vi "Car Wash.vi"() -> ()   [LabVIEW 2013]
doc: "THis VI is a simulation of automated car wash controller.\nthe user can interact with the controls and indicator and select the car wash option and simulates the travel of the vehicle in the car wash.\n\nThe controller can perform these operation.\n- Indicate the car wash LED if the car wash is vacant or wash in progress.\n- Allow the user to select Wash option.\n- On pressing start the washing process will begin.\n- Indicator indicates the current wash process and display the elapsed time on indicator\n- Turn On the vehicle out of position LED and pause the elapsed time if the vehicle moves from its place \n during a cycle."
uses:
  Controls/Car Wash Indicators.ctl
  Controls/Wash Options.ctl
  Controls/Car wash cmd data cluster.ctl
  Controls/Car Wash States.ctl
  Controls/fgv.ctl
panel:
  in  "Start":bool
  out "Elapsed Time":dbl format="%0.2f"
  in  "stop":bool
  out "Wash Entry":bool
  in  "Wash Options":T1
  in  "Car Position Slider":u8(slide) max=3 scale=0.0..4.0
  out "Car Wash Indicators":T2
  # "Entry Console"
  # "Car Wash Display"
  # "Car Position Simulation"
  # "Pre-Soak\nH-P Wash\nL-P Wax\nSpot Free Rinse"
  # "Underbody Wash\nBug Remover"
  # "Tire Shine\nAir Dry"
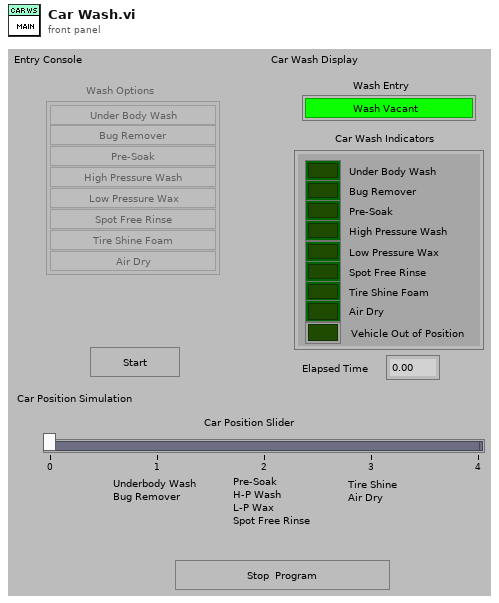
[diagram p1: front panel]
types:
  T1 = typedef "Wash Options.ctl" = cluster{"Underbody Wash":bool, "Bug Remover":bool, "Pre-Soak":bool, "High Pressure Wash":bool, "Low Pressure Wax":bool, "Spot Free Rinse":bool, "Tire Shine Foam":bool, "Air Dry":bool}
  T2 = typedef "Car Wash Indicators.ctl" = cluster{"Under Body Wash":bool, "Bug Remover":bool, "Pre-Soak":bool, "High Pressure Wash":bool, "Low Pressure Wax":bool, "Spot Free Rinse":bool, "Tire Shine Foam":bool, "Air Dry":bool, "Vehicle Out of Position":bool}
  T3 = typedef "Car wash cmd data cluster.ctl" = cluster{"Command":T4, "Data":variant}
  T4 = typedef "Car Wash States.ctl" = enum16{"Initialize", "Start1", "Start", "Underbody Wash", "Bug Remover", "Pre-Soak", "High Pressure Wash", "Low pressure wash", "Spot free Rinse", "Tire Shine Foam", "Air Dry", "Stop"}
  T5 = cluster{"Car Wash Indicators":T2, "Wash Entry":bool, "Elapsed TIme":dbl}
  T6 = enum8{"Enabled", "Disabled", "Disabled and Grayed Out"}
  T7 = typedef "fgv.ctl" = enum16{"Set Car Pos.", "Get Car Pos."}
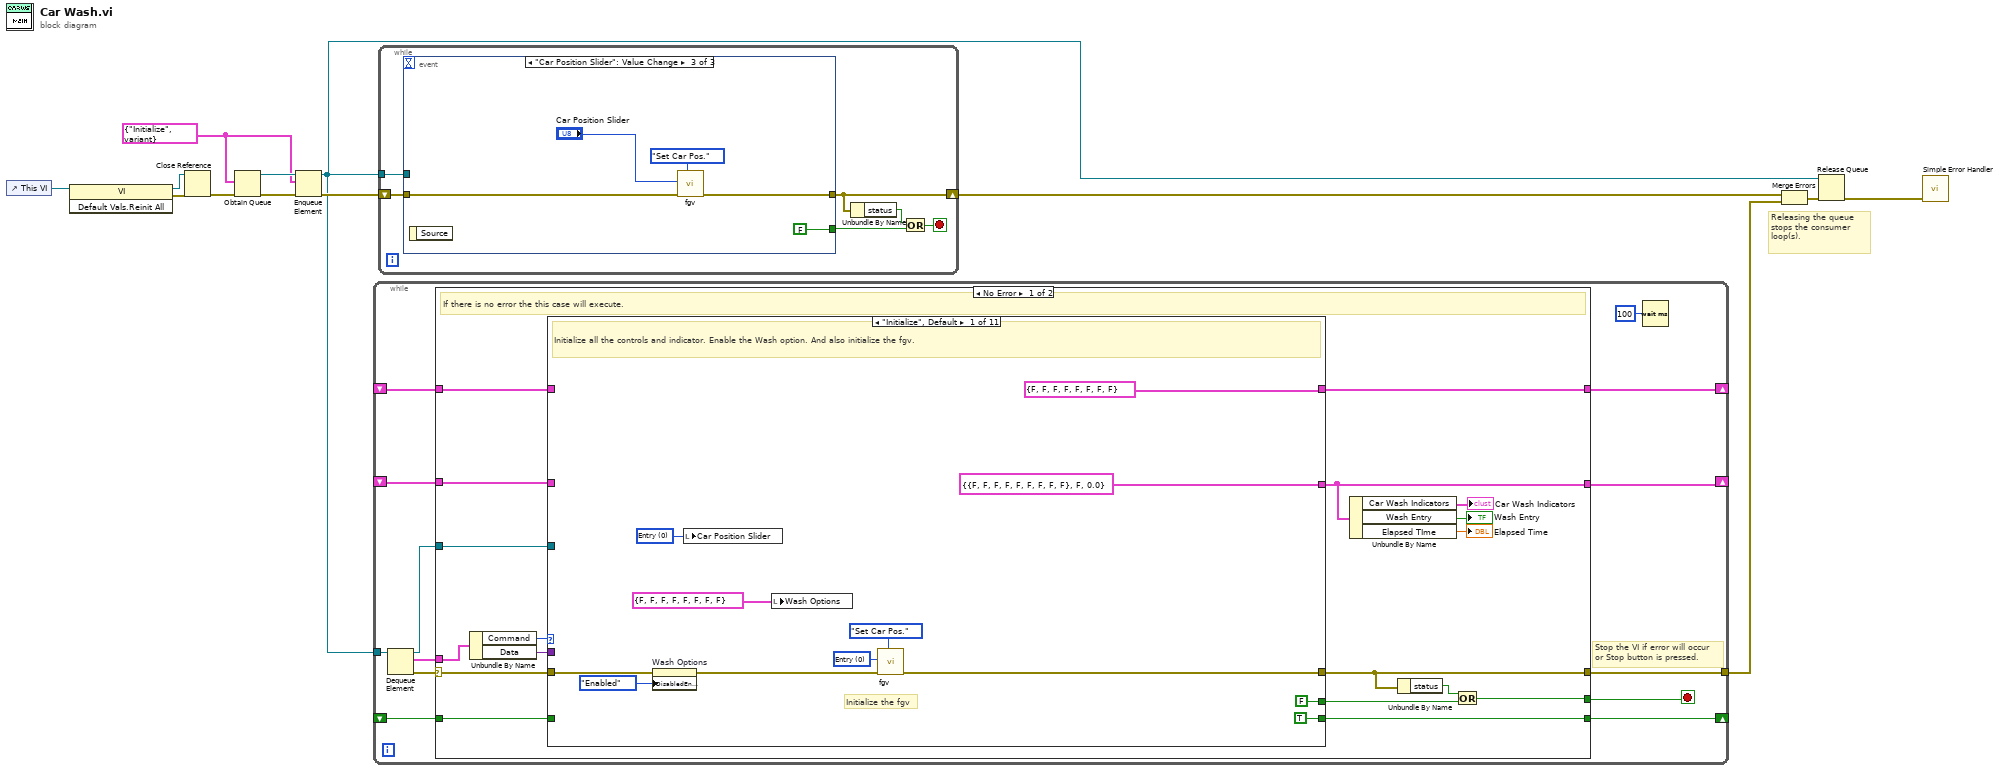
[diagram p0: block diagram]
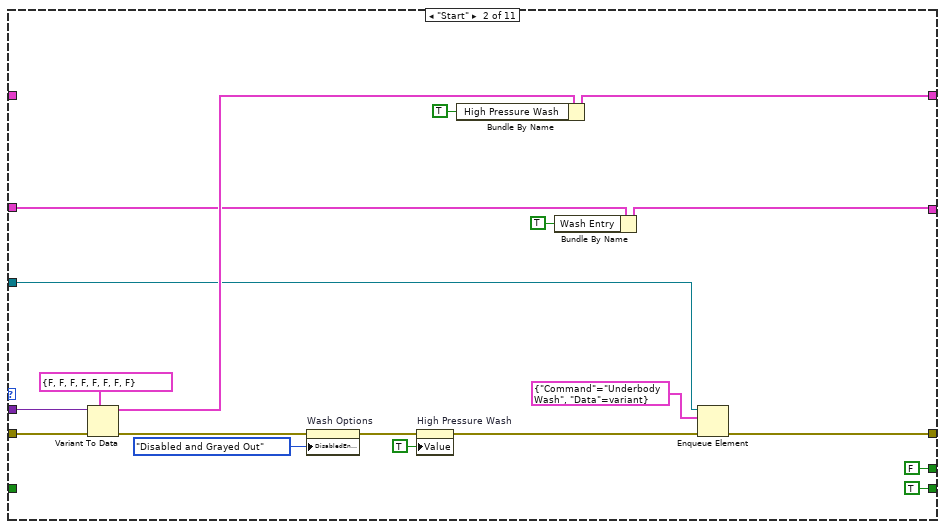
[diagram p2: hidden frame]
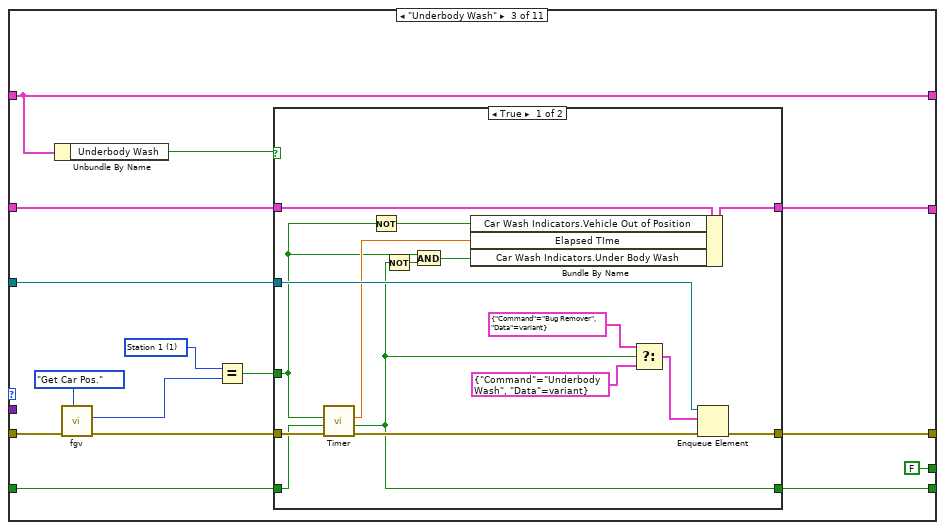
[diagram p3: hidden frame]
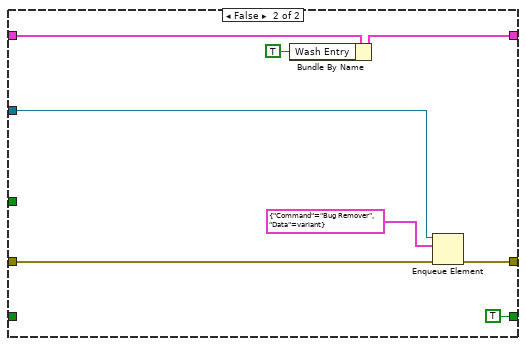
[diagram p4: hidden frame]
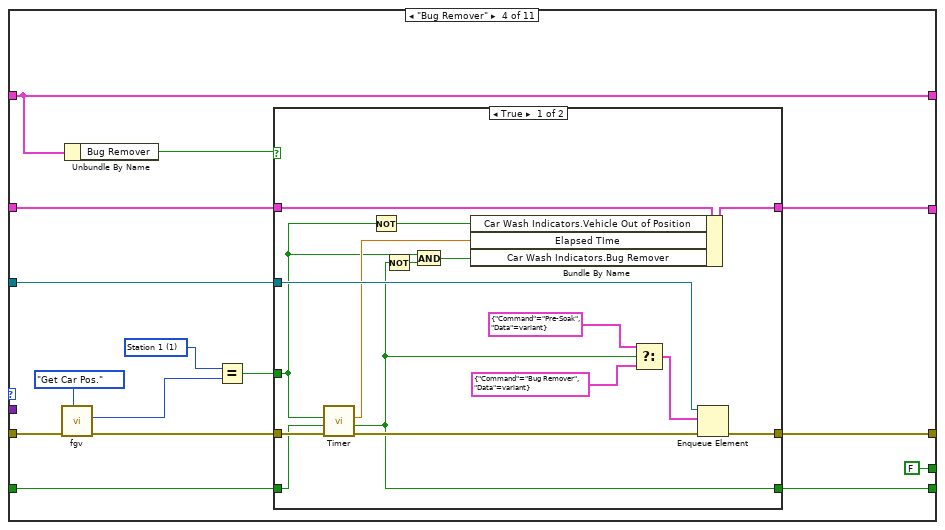
[diagram p5: hidden frame]
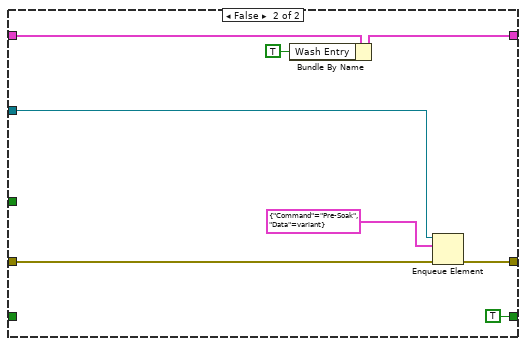
[diagram p6: hidden frame]
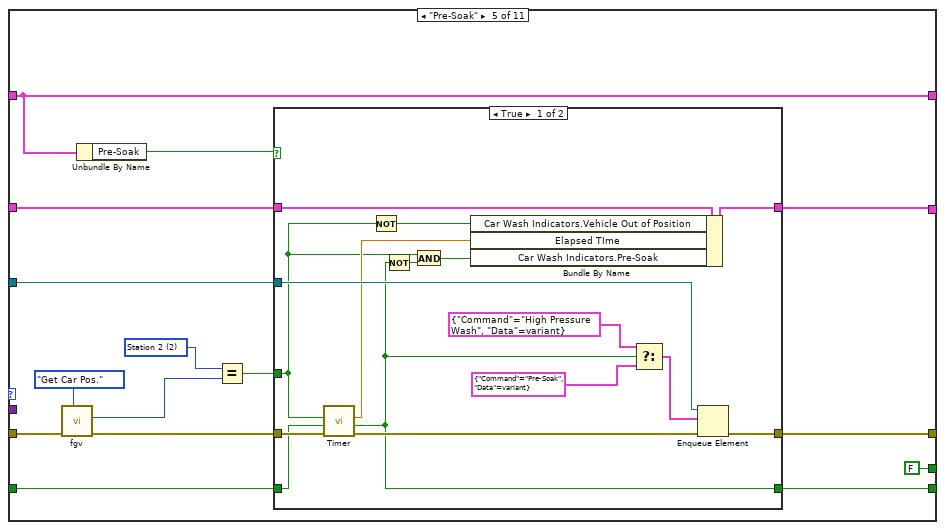
[diagram p7: hidden frame]
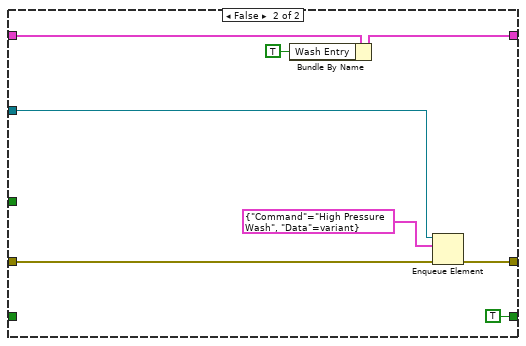
[diagram p8: hidden frame]
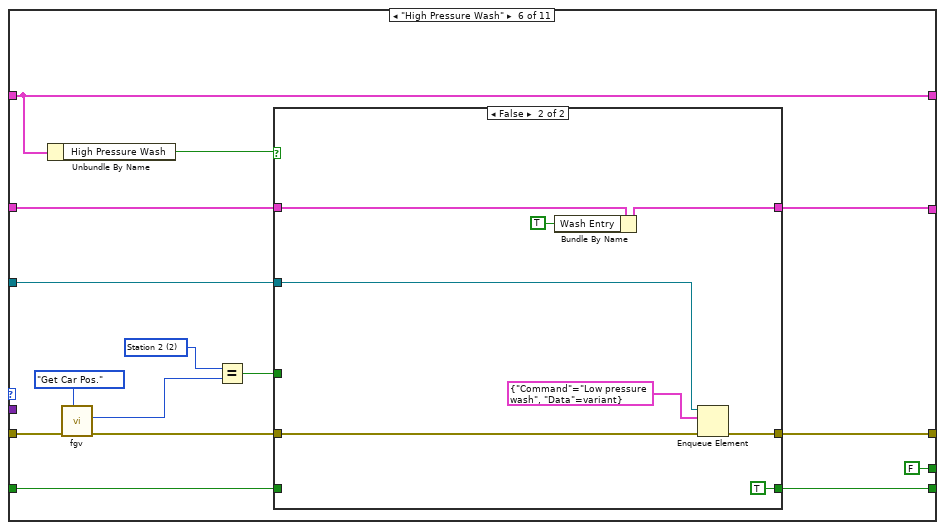
[diagram p9: hidden frame]
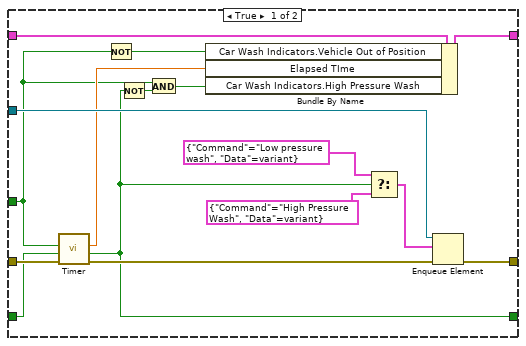
[diagram p10: hidden frame]
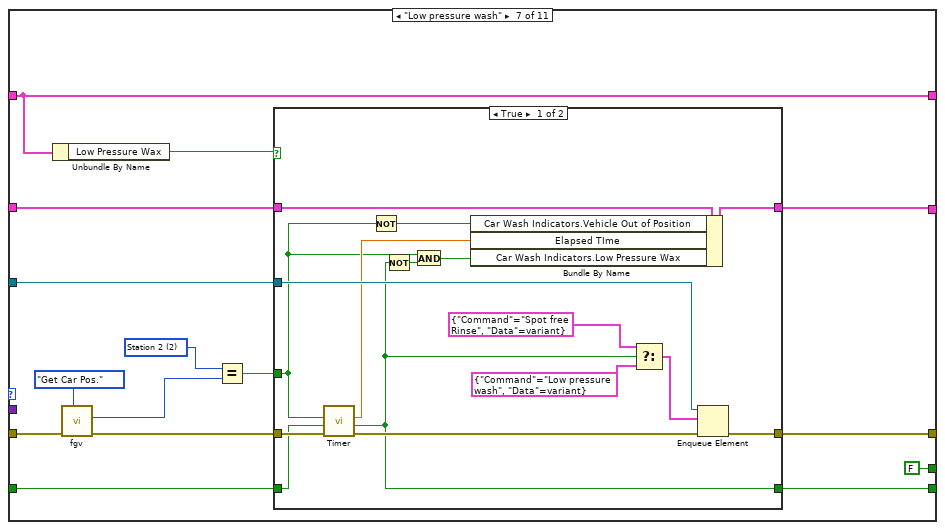
[diagram p11: hidden frame]
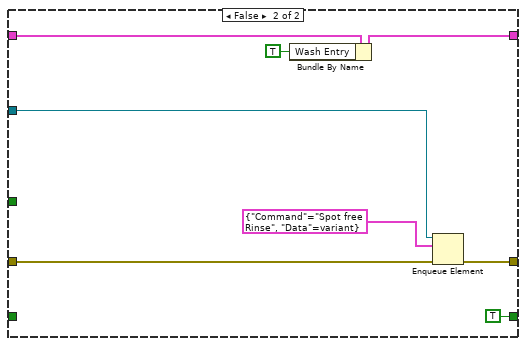
[diagram p12: hidden frame]
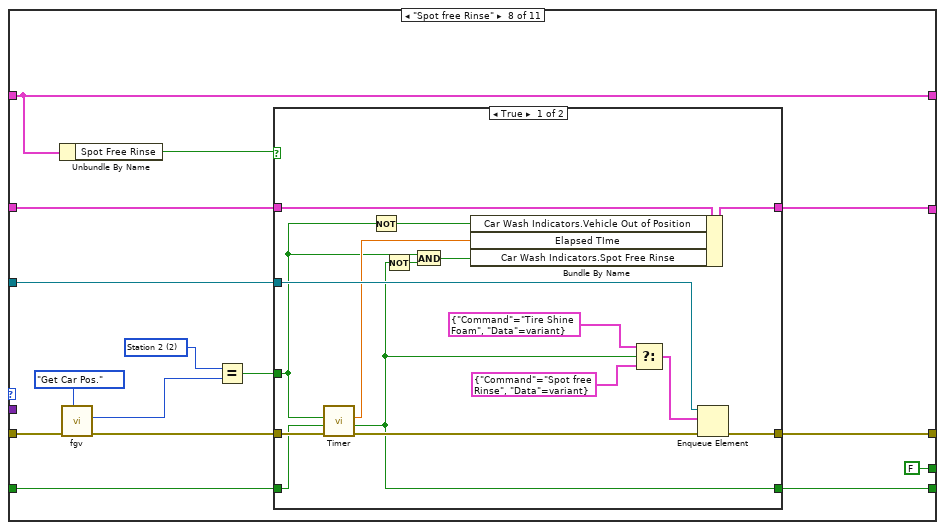
[diagram p13: hidden frame]
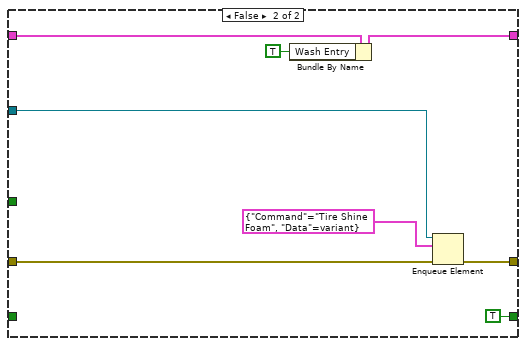
[diagram p14: hidden frame]
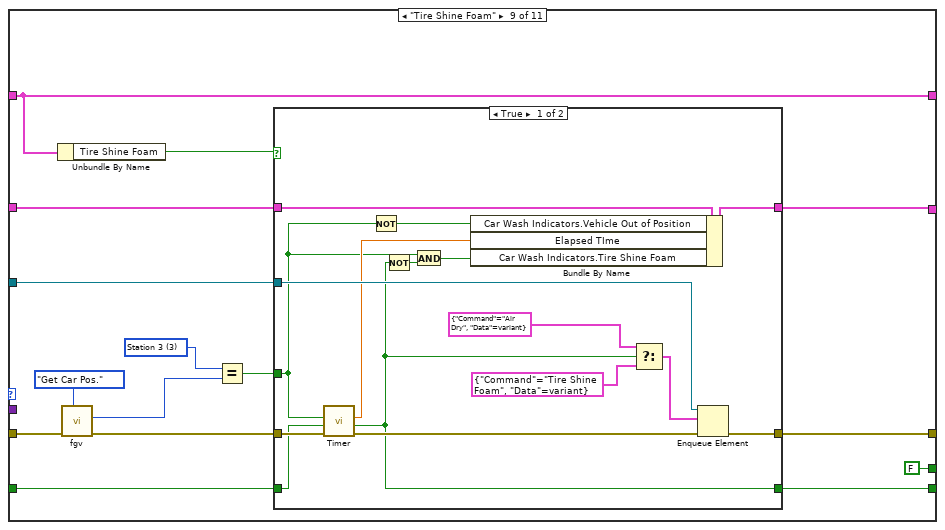
[diagram p15: hidden frame]
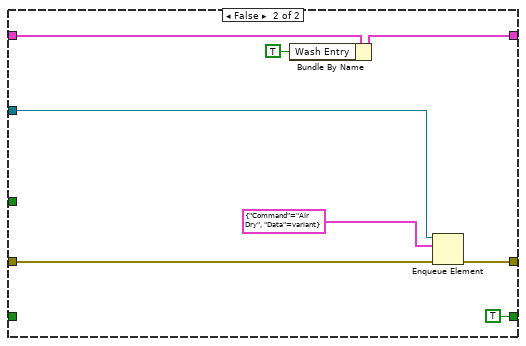
[diagram p16: hidden frame]
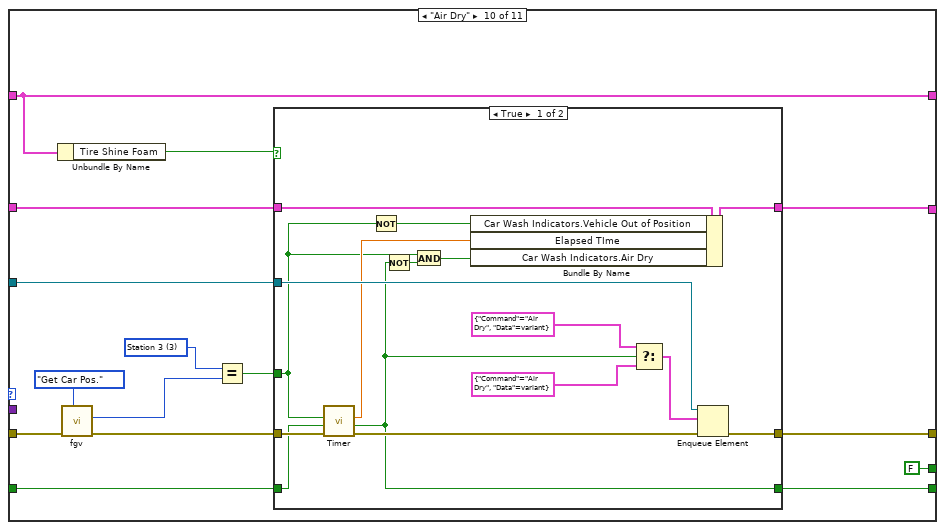
[diagram p17: hidden frame]
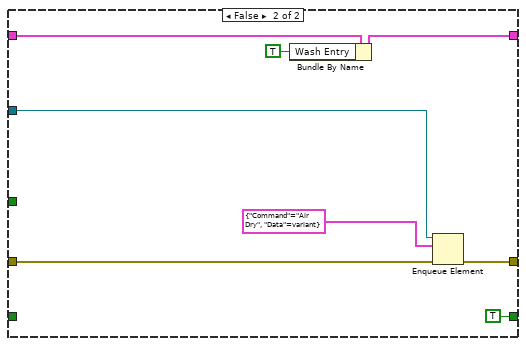
[diagram p18: hidden frame]
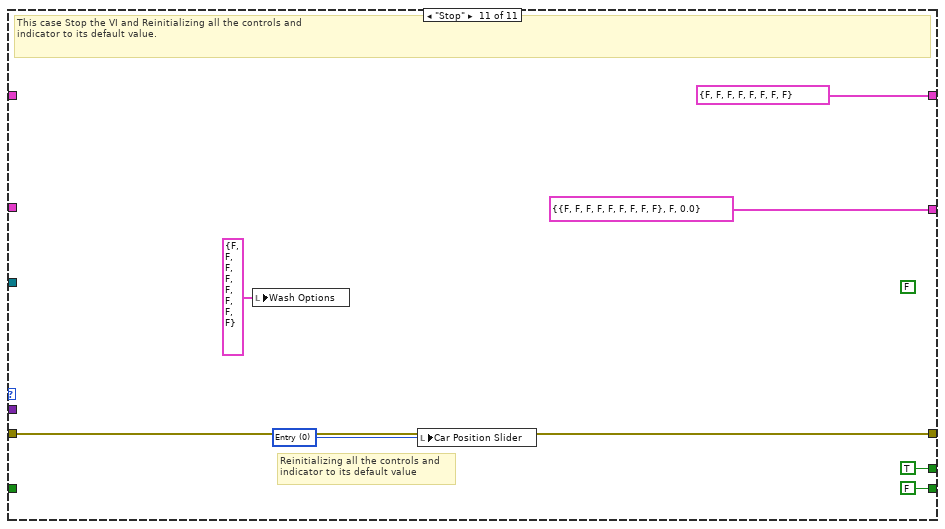
[diagram p19: hidden frame]
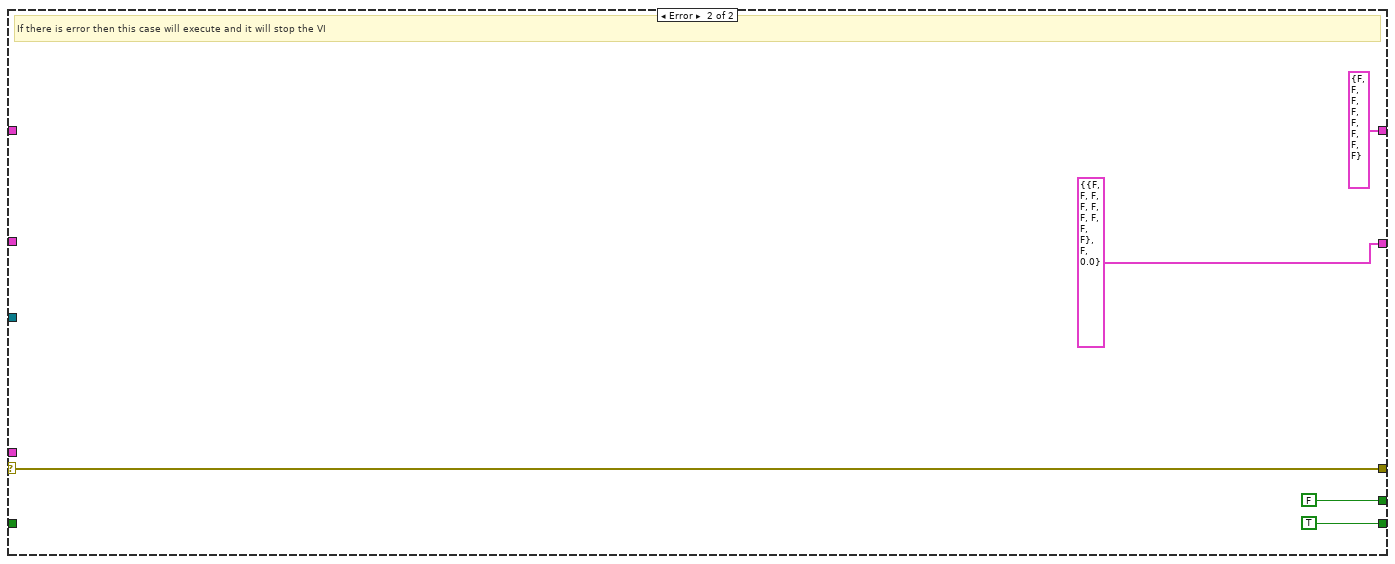
[diagram p20: hidden frame]
diagram:
  w1 = T3 {"Command"=enum."Initialize", "Data"=variant} ("Car wash cmd data cluster")
  # "Releasing the queue stops the consumer loop(s)."
  n1 = control-ref of="This VI"() -> (w9:refnum<vi>)
  n2 = invoke class="VI" method="Default Vals.Reinit All"(reference=w9) -> (reference out=w7:refnum<vi>, error out=w8:errorcluster)  [unwired: 2 in, 1 out]
  n3 = Close Reference(reference=w7, error in (no error)=w8) -> (error out=w6:errorcluster)
  n4 = Obtain Queue(element data type=w1, error in (no error)=w6) -> (queue out=w13:refnum<queue>, error out=w12:errorcluster)  [unwired: 3 in, 1 out]
  n5 = Enqueue Element(queue=w13, element=w1, error in (no error)=w12) -> (queue out=w10:refnum<queue>, error out=w11:errorcluster)  [unwired: 1 in, 1 out]
  n6 = while {
    tunnel: w10 -> [w26]
    tunnel: [w23] -> w3
    shift-right: [w22] -> _
    shift-left: _ -> [w21]
    shift-right: [w19] -> _
    shift-left: _ -> [w18]
    shift-right: [w16] -> _
    shift-left: _ -> [w14]
    stop <- w17 stop-if-true
    # "Stop the VI if error will occur \nor Stop button is pressed."
    n7 = Dequeue Element(queue=w26) -> (queue out=w15:refnum<queue>, element=w24:T3, error out=w25:errorcluster)  [unwired: 2 in, 1 out]
    n8 = case shown="No Error" w25 {
      selector: w25 -> [w42 w399]
      tunnel: w24 -> [w44 _]
      tunnel: [w36 w399] -> w23
      tunnel: [w35 FALSE] -> w17
      tunnel: [w41 TRUE ("Elapsed?")] -> w22
      tunnel: w21 -> [w40 _]
      tunnel: [w33 T5 {"Car Wash Indicators"={"Under Body Wash"=FALSE, "Bug Remover"=FALSE, "Pre-Soak"=FALSE, "High Pressure Wash"=FALSE, "Low Pressure Wax"=FALSE, "Spot Free Rinse"=FALSE, "Tire Shine Foam"=FALSE, "Air Dry"=FALSE, "Vehicle Out of Position"=FALSE}, "Wash Entry"=FALSE, "Elapsed TIme"=0.0}] -> w19
      tunnel: w18 -> [w39 _]
      tunnel: [w29 T1 {"Underbody Wash"=FALSE, "Bug Remover"=FALSE, "Pre-Soak"=FALSE, "High Pressure Wash"=FALSE, "Low Pressure Wax"=FALSE, "Spot Free Rinse"=FALSE, "Tire Shine Foam"=FALSE, "Air Dry"=FALSE} ("Wash Options")] -> w16
      tunnel: w15 -> [w28 _]
      tunnel: w14 -> [w27 _]
      frame No Error {
        # "If there is no error the this case will execute."
        n9 = Unbundle By Name(w44) -> ("Command"=w43:T4, "Data"=w30:variant)
        n10 = case shown="\"Initialize\", Default" w43 {
          tunnel: w42 -> [w51 w75 w85 w124 w163 w202 w241 w280 w319 w358 w394]
          tunnel: [w54 w58 w87 w126 w165 w204 w243 w282 w321 w360 w394] -> w36
          tunnel: [FALSE FALSE FALSE FALSE FALSE FALSE FALSE FALSE FALSE FALSE TRUE] -> w37
          tunnel: [TRUE TRUE ("Elapsed?") w76 w115 w154 w193 w232 w271 w310 w349 FALSE ("Elapsed?")] -> w41
          tunnel: w40 -> [_ _ w77 w116 w155 w194 w233 w272 w311 w350 _]
          tunnel: [T5 {"Car Wash Indicators"={"Under Body Wash"=FALSE, "Bug Remover"=FALSE, "Pre-Soak"=FALSE, "High Pressure Wash"=FALSE, "Low Pressure Wax"=FALSE, "Spot Free Rinse"=FALSE, "Tire Shine Foam"=FALSE, "Air Dry"=FALSE, "Vehicle Out of Position"=FALSE}, "Wash Entry"=FALSE, "Elapsed TIme"=0.0} w65 w88 w127 w166 w205 w244 w283 w322 w361 T5 {"Car Wash Indicators"={"Under Body Wash"=FALSE, "Bug Remover"=FALSE, "Pre-Soak"=FALSE, "High Pressure Wash"=FALSE, "Low Pressure Wax"=FALSE, "Spot Free Rinse"=FALSE, "Tire Shine Foam"=FALSE, "Air Dry"=FALSE, "Vehicle Out of Position"=FALSE}, "Wash Entry"=FALSE, "Elapsed TIme"=0.0}] -> w33
          tunnel: w39 -> [_ w66 w89 w128 w167 w206 w245 w284 w323 w362 _]
          tunnel: w30 -> [_ w74 _ _ _ _ _ _ _ _ _]
          tunnel: [T1 {"Underbody Wash"=FALSE, "Bug Remover"=FALSE, "Pre-Soak"=FALSE, "High Pressure Wash"=FALSE, "Low Pressure Wax"=FALSE, "Spot Free Rinse"=FALSE, "Tire Shine Foam"=FALSE, "Air Dry"=FALSE} ("Wash Options") w71 w80 w119 w158 w197 w236 w275 w314 w353 T1 {"Underbody Wash"=FALSE, "Bug Remover"=FALSE, "Pre-Soak"=FALSE, "High Pressure Wash"=FALSE, "Low Pressure Wax"=FALSE, "Spot Free Rinse"=FALSE, "Tire Shine Foam"=FALSE, "Air Dry"=FALSE} ("Wash Options")] -> w29
          tunnel: w28 -> [_ w57 w86 w125 w164 w203 w242 w281 w320 w359 _]
          tunnel: w27 -> [_ _ w80 w119 w158 w197 w236 w275 w314 w353 _]
          frame "Initialize", Default {
            w45 = u8 0 items=["Entry", "Station 1", "Station 2", "Station 3", "Exit"] ("Car Position Slider")
            w48 = u8 0 items=["Entry", "Station 1", "Station 2", "Station 3", "Exit"] ("Car Position Slider")
            # "Initialize the fgv"
            # "Initialize all the controls and indicator. Enable the Wash option. And also initialize the fgv."
            n11 = property on="Wash Options" class="Clust (strict)"(error in=w51, "DisabledEnum"=T6."Enabled" ("Disabled")) -> (error out=w50:errorcluster)  [unwired: 1 in, 1 out]
            n12 = local write "Car Position Slider"(w48) -> ()
            n13 = local write "Wash Options"(T1 {"Underbody Wash"=FALSE, "Bug Remover"=FALSE, "Pre-Soak"=FALSE, "High Pressure Wash"=FALSE, "Low Pressure Wax"=FALSE, "Spot Free Rinse"=FALSE, "Tire Shine Foam"=FALSE, "Air Dry"=FALSE} ("Wash Options")) -> ()
            n14 = call "fgv.vi"("Command"=fgv."Set Car Pos.", "error in (no error)"=w50, "Car Position Slider"=w45) -> ("error out"=w54:errorcluster)  [unwired: 7 in, 1 out]
          }
          frame "Start" {
            n15 = Variant To Data(error in=w75, type=T1 {"Underbody Wash"=FALSE, "Bug Remover"=FALSE, "Pre-Soak"=FALSE, "High Pressure Wash"=FALSE, "Low Pressure Wax"=FALSE, "Spot Free Rinse"=FALSE, "Tire Shine Foam"=FALSE, "Air Dry"=FALSE} ("Wash Options"), Variant=w74) -> (data=w73:T1, error out=w67:errorcluster)
            n16 = property on="Wash Options" class="Clust (strict)"(error in=w67, "DisabledEnum"=T6."Disabled and Grayed Out" ("Disabled")) -> (error out=w62:errorcluster)  [unwired: 1 in, 1 out]
            n17 = property on="High Pressure Wash" class="Bool (strict)"(error in=w62, "Value"=TRUE) -> (error out=w59:errorcluster)  [unwired: 1 in, 1 out]
            n18 = Bundle By Name(cluster=w73, "High Pressure Wash"=TRUE) -> (w71:T1)
            n19 = Bundle By Name(cluster=w66, "Wash Entry"=TRUE) -> (w65:T5)
            n20 = Enqueue Element(queue=w57, element=T3 {"Command"=enum."Underbody Wash", "Data"=variant} ("Car wash cmd data cluster"), error in (no error)=w59) -> (error out=w58:errorcluster)  [unwired: 1 in, 2 out]
          }
          frame "Underbody Wash" {
            w81 = u8 1 items=["Entry", "Station 1", "Station 2", "Station 3", "Exit"] ("Car Position Slider")
            n21 = Unbundle By Name(w80) -> ("Underbody Wash"=w79:bool)
            n22 = call "fgv.vi"("Command"=fgv."Get Car Pos.", "error in (no error)"=w85) -> ("error out"=w84:errorcluster, "Car Position Slider 2"=w82:u8)  [unwired: 8 in]
            n23 = Equal?(x=w81, y=w82) -> (x = y?=w78:bool)
            n24 = case shown="True" w79 {
              tunnel: w89 -> [w106 w114]
              tunnel: [w105 w113] -> w88
              tunnel: [w104 w110] -> w87
              tunnel: w86 -> [w103 w109]
              tunnel: w84 -> [w102 w108]
              tunnel: w78 -> [w91 _]
              tunnel: w77 -> [w100 _]
              tunnel: [w93 TRUE ("Elapsed?")] -> w76
              frame True {
                n25 = call "Timer.vi"("error in (no error)"=w102, "Reset"=w100, "Pause"=w91) -> ("error out"=w101:errorcluster, "Elapsed?"=w93:bool, "Elapsed TIme"=w96:dbl)  [unwired: 6 in]
                n26 = Not(x=w91) -> (.not. x?=w95:bool)
                n27 = Not(x=w93) -> (.not. x?=w92:bool)
                n28 = And(x=w91, y=w92) -> (x .and. y?=w94:bool)
                n29 = Bundle By Name(cluster=w106, "Car Wash Indicators.Vehicle Out of Position"=w95, "Elapsed TIme"=w96, "Car Wash Indicators.Under Body Wash"=w94) -> (w105:T5)
                n30 = Select(t=T3 {"Command"=enum."Bug Remover", "Data"=variant} ("Car wash cmd data cluster"), s=w93, f=T3 {"Command"=enum."Underbody Wash", "Data"=variant}) -> (s? t:f=w97:T3)
                n31 = Enqueue Element(queue=w103, element=w97, error in (no error)=w101) -> (error out=w104:errorcluster)  [unwired: 1 in, 2 out]
              }
              frame False {
                n32 = Bundle By Name(cluster=w114, "Wash Entry"=TRUE) -> (w113:T5)
                n33 = Enqueue Element(queue=w109, element=T3 {"Command"=enum."Bug Remover", "Data"=variant} ("Car wash cmd data cluster"), error in (no error)=w108) -> (error out=w110:errorcluster)  [unwired: 1 in, 2 out]
              }
            }
          }
          frame "Bug Remover" {
            w120 = u8 1 items=["Entry", "Station 1", "Station 2", "Station 3", "Exit"] ("Car Position Slider")
            n34 = call "fgv.vi"("Command"=fgv."Get Car Pos.", "error in (no error)"=w124) -> ("error out"=w123:errorcluster, "Car Position Slider 2"=w121:u8)  [unwired: 8 in]
            n35 = Unbundle By Name(w119) -> ("Bug Remover"=w118:bool)
            n36 = Equal?(x=w120, y=w121) -> (x = y?=w117:bool)
            n37 = case shown="True" w118 {
              tunnel: w128 -> [w145 w153]
              tunnel: [w144 w152] -> w127
              tunnel: [w143 w149] -> w126
              tunnel: w125 -> [w142 w148]
              tunnel: w123 -> [w141 w147]
              tunnel: w117 -> [w130 _]
              tunnel: w116 -> [w139 _]
              tunnel: [w132 TRUE ("Elapsed?")] -> w115
              frame True {
                n38 = call "Timer.vi"("error in (no error)"=w141, "Reset"=w139, "Pause"=w130) -> ("error out"=w140:errorcluster, "Elapsed?"=w132:bool, "Elapsed TIme"=w135:dbl)  [unwired: 6 in]
                n39 = Not(x=w130) -> (.not. x?=w134:bool)
                n40 = Not(x=w132) -> (.not. x?=w131:bool)
                n41 = And(x=w130, y=w131) -> (x .and. y?=w133:bool)
                n42 = Bundle By Name(cluster=w145, "Car Wash Indicators.Vehicle Out of Position"=w134, "Elapsed TIme"=w135, "Car Wash Indicators.Bug Remover"=w133) -> (w144:T5)
                n43 = Select(t=T3 {"Command"=enum."Pre-Soak", "Data"=variant} ("Car wash cmd data cluster"), s=w132, f=T3 {"Command"=enum."Bug Remover", "Data"=variant}) -> (s? t:f=w136:T3)
                n44 = Enqueue Element(queue=w142, element=w136, error in (no error)=w140) -> (error out=w143:errorcluster)  [unwired: 1 in, 2 out]
              }
              frame False {
                n45 = Bundle By Name(cluster=w153, "Wash Entry"=TRUE) -> (w152:T5)
                n46 = Enqueue Element(queue=w148, element=T3 {"Command"=enum."Pre-Soak", "Data"=variant} ("Car wash cmd data cluster"), error in (no error)=w147) -> (error out=w149:errorcluster)  [unwired: 1 in, 2 out]
              }
            }
          }
          frame "Pre-Soak" {
            w159 = u8 2 items=["Entry", "Station 1", "Station 2", "Station 3", "Exit"] ("Car Position Slider")
            n47 = call "fgv.vi"("Command"=fgv."Get Car Pos.", "error in (no error)"=w163) -> ("error out"=w162:errorcluster, "Car Position Slider 2"=w160:u8)  [unwired: 8 in]
            n48 = Unbundle By Name(w158) -> ("Pre-Soak"=w157:bool)
            n49 = Equal?(x=w159, y=w160) -> (x = y?=w156:bool)
            n50 = case shown="True" w157 {
              tunnel: w167 -> [w184 w192]
              tunnel: [w183 w191] -> w166
              tunnel: [w182 w188] -> w165
              tunnel: w164 -> [w181 w187]
              tunnel: w162 -> [w180 w186]
              tunnel: w156 -> [w169 _]
              tunnel: w155 -> [w178 _]
              tunnel: [w171 TRUE ("Elapsed?")] -> w154
              frame True {
                n51 = call "Timer.vi"("error in (no error)"=w180, "Reset"=w178, "Pause"=w169) -> ("error out"=w179:errorcluster, "Elapsed?"=w171:bool, "Elapsed TIme"=w174:dbl)  [unwired: 6 in]
                n52 = Not(x=w169) -> (.not. x?=w173:bool)
                n53 = Not(x=w171) -> (.not. x?=w170:bool)
                n54 = And(x=w169, y=w170) -> (x .and. y?=w172:bool)
                n55 = Bundle By Name(cluster=w184, "Car Wash Indicators.Vehicle Out of Position"=w173, "Elapsed TIme"=w174, "Car Wash Indicators.Pre-Soak"=w172) -> (w183:T5)
                n56 = Select(t=T3 {"Command"=enum."High Pressure Wash", "Data"=variant} ("Car wash cmd data cluster"), s=w171, f=T3 {"Command"=enum."Pre-Soak", "Data"=variant}) -> (s? t:f=w175:T3)
                n57 = Enqueue Element(queue=w181, element=w175, error in (no error)=w179) -> (error out=w182:errorcluster)  [unwired: 1 in, 2 out]
              }
              frame False {
                n58 = Bundle By Name(cluster=w192, "Wash Entry"=TRUE) -> (w191:T5)
                n59 = Enqueue Element(queue=w187, element=T3 {"Command"=enum."High Pressure Wash", "Data"=variant} ("Car wash cmd data cluster"), error in (no error)=w186) -> (error out=w188:errorcluster)  [unwired: 1 in, 2 out]
              }
            }
          }
          frame "High Pressure Wash" {
            w198 = u8 2 items=["Entry", "Station 1", "Station 2", "Station 3", "Exit"] ("Car Position Slider")
            n60 = Unbundle By Name(w197) -> ("High Pressure Wash"=w196:bool)
            n61 = call "fgv.vi"("Command"=fgv."Get Car Pos.", "error in (no error)"=w202) -> ("error out"=w201:errorcluster, "Car Position Slider 2"=w199:u8)  [unwired: 8 in]
            n62 = Equal?(x=w198, y=w199) -> (x = y?=w195:bool)
            n63 = case shown="False" w196 {
              tunnel: w206 -> [w223 w231]
              tunnel: [w222 w230] -> w205
              tunnel: [w221 w227] -> w204
              tunnel: w203 -> [w220 w226]
              tunnel: w201 -> [w219 w225]
              tunnel: w195 -> [w208 _]
              tunnel: w194 -> [w217 _]
              tunnel: [w210 TRUE ("Elapsed?")] -> w193
              frame True {
                n64 = call "Timer.vi"("error in (no error)"=w219, "Reset"=w217, "Pause"=w208) -> ("error out"=w218:errorcluster, "Elapsed?"=w210:bool, "Elapsed TIme"=w213:dbl)  [unwired: 6 in]
                n65 = Not(x=w208) -> (.not. x?=w212:bool)
                n66 = Not(x=w210) -> (.not. x?=w209:bool)
                n67 = And(x=w208, y=w209) -> (x .and. y?=w211:bool)
                n68 = Bundle By Name(cluster=w223, "Car Wash Indicators.Vehicle Out of Position"=w212, "Elapsed TIme"=w213, "Car Wash Indicators.High Pressure Wash"=w211) -> (w222:T5)
                n69 = Select(t=T3 {"Command"=enum."Low pressure wash", "Data"=variant} ("Car wash cmd data cluster"), s=w210, f=T3 {"Command"=enum."High Pressure Wash", "Data"=variant}) -> (s? t:f=w214:T3)
                n70 = Enqueue Element(queue=w220, element=w214, error in (no error)=w218) -> (error out=w221:errorcluster)  [unwired: 1 in, 2 out]
              }
              frame False {
                n71 = Bundle By Name(cluster=w231, "Wash Entry"=TRUE) -> (w230:T5)
                n72 = Enqueue Element(queue=w226, element=T3 {"Command"=enum."Low pressure wash", "Data"=variant} ("Car wash cmd data cluster"), error in (no error)=w225) -> (error out=w227:errorcluster)  [unwired: 1 in, 2 out]
              }
            }
          }
          frame "Low pressure wash" {
            w237 = u8 2 items=["Entry", "Station 1", "Station 2", "Station 3", "Exit"] ("Car Position Slider")
            n73 = Unbundle By Name(w236) -> ("Low Pressure Wax"=w235:bool)
            n74 = call "fgv.vi"("Command"=fgv."Get Car Pos.", "error in (no error)"=w241) -> ("error out"=w240:errorcluster, "Car Position Slider 2"=w238:u8)  [unwired: 8 in]
            n75 = Equal?(x=w237, y=w238) -> (x = y?=w234:bool)
            n76 = case shown="True" w235 {
              tunnel: w245 -> [w262 w270]
              tunnel: [w261 w269] -> w244
              tunnel: [w260 w266] -> w243
              tunnel: w242 -> [w259 w265]
              tunnel: w240 -> [w258 w264]
              tunnel: w234 -> [w247 _]
              tunnel: w233 -> [w256 _]
              tunnel: [w249 TRUE ("Elapsed?")] -> w232
              frame True {
                n77 = call "Timer.vi"("error in (no error)"=w258, "Reset"=w256, "Pause"=w247) -> ("error out"=w257:errorcluster, "Elapsed?"=w249:bool, "Elapsed TIme"=w252:dbl)  [unwired: 6 in]
                n78 = Not(x=w247) -> (.not. x?=w251:bool)
                n79 = Not(x=w249) -> (.not. x?=w248:bool)
                n80 = And(x=w247, y=w248) -> (x .and. y?=w250:bool)
                n81 = Bundle By Name(cluster=w262, "Car Wash Indicators.Vehicle Out of Position"=w251, "Elapsed TIme"=w252, "Car Wash Indicators.Low Pressure Wax"=w250) -> (w261:T5)
                n82 = Select(t=T3 {"Command"=enum."Spot free Rinse", "Data"=variant} ("Car wash cmd data cluster"), s=w249, f=T3 {"Command"=enum."Low pressure wash", "Data"=variant}) -> (s? t:f=w253:T3)
                n83 = Enqueue Element(queue=w259, element=w253, error in (no error)=w257) -> (error out=w260:errorcluster)  [unwired: 1 in, 2 out]
              }
              frame False {
                n84 = Bundle By Name(cluster=w270, "Wash Entry"=TRUE) -> (w269:T5)
                n85 = Enqueue Element(queue=w265, element=T3 {"Command"=enum."Spot free Rinse", "Data"=variant} ("Car wash cmd data cluster"), error in (no error)=w264) -> (error out=w266:errorcluster)  [unwired: 1 in, 2 out]
              }
            }
          }
          frame "Spot free Rinse" {
            w276 = u8 2 items=["Entry", "Station 1", "Station 2", "Station 3", "Exit"] ("Car Position Slider")
            n86 = Unbundle By Name(w275) -> ("Spot Free Rinse"=w274:bool)
            n87 = call "fgv.vi"("Command"=fgv."Get Car Pos.", "error in (no error)"=w280) -> ("error out"=w279:errorcluster, "Car Position Slider 2"=w277:u8)  [unwired: 8 in]
            n88 = Equal?(x=w276, y=w277) -> (x = y?=w273:bool)
            n89 = case shown="True" w274 {
              tunnel: w284 -> [w301 w309]
              tunnel: [w300 w308] -> w283
              tunnel: [w299 w305] -> w282
              tunnel: w281 -> [w298 w304]
              tunnel: w279 -> [w297 w303]
              tunnel: w273 -> [w286 _]
              tunnel: w272 -> [w295 _]
              tunnel: [w288 TRUE ("Elapsed?")] -> w271
              frame True {
                n90 = call "Timer.vi"("error in (no error)"=w297, "Reset"=w295, "Pause"=w286) -> ("error out"=w296:errorcluster, "Elapsed?"=w288:bool, "Elapsed TIme"=w291:dbl)  [unwired: 6 in]
                n91 = Not(x=w286) -> (.not. x?=w290:bool)
                n92 = Not(x=w288) -> (.not. x?=w287:bool)
                n93 = And(x=w286, y=w287) -> (x .and. y?=w289:bool)
                n94 = Bundle By Name(cluster=w301, "Car Wash Indicators.Vehicle Out of Position"=w290, "Elapsed TIme"=w291, "Car Wash Indicators.Spot Free Rinse"=w289) -> (w300:T5)
                n95 = Select(t=T3 {"Command"=enum."Tire Shine Foam", "Data"=variant} ("Car wash cmd data cluster"), s=w288, f=T3 {"Command"=enum."Spot free Rinse", "Data"=variant}) -> (s? t:f=w292:T3)
                n96 = Enqueue Element(queue=w298, element=w292, error in (no error)=w296) -> (error out=w299:errorcluster)  [unwired: 1 in, 2 out]
              }
              frame False {
                n97 = Bundle By Name(cluster=w309, "Wash Entry"=TRUE) -> (w308:T5)
                n98 = Enqueue Element(queue=w304, element=T3 {"Command"=enum."Tire Shine Foam", "Data"=variant} ("Car wash cmd data cluster"), error in (no error)=w303) -> (error out=w305:errorcluster)  [unwired: 1 in, 2 out]
              }
            }
          }
          frame "Tire Shine Foam" {
            w315 = u8 3 items=["Entry", "Station 1", "Station 2", "Station 3", "Exit"] ("Car Position Slider")
            n99 = Unbundle By Name(w314) -> ("Tire Shine Foam"=w313:bool)
            n100 = call "fgv.vi"("Command"=fgv."Get Car Pos.", "error in (no error)"=w319) -> ("error out"=w318:errorcluster, "Car Position Slider 2"=w316:u8)  [unwired: 8 in]
            n101 = Equal?(x=w315, y=w316) -> (x = y?=w312:bool)
            n102 = case shown="True" w313 {
              tunnel: w323 -> [w340 w348]
              tunnel: [w339 w347] -> w322
              tunnel: [w338 w344] -> w321
              tunnel: w320 -> [w337 w343]
              tunnel: w318 -> [w336 w342]
              tunnel: w312 -> [w325 _]
              tunnel: w311 -> [w334 _]
              tunnel: [w327 TRUE ("Elapsed?")] -> w310
              frame True {
                n103 = call "Timer.vi"("error in (no error)"=w336, "Reset"=w334, "Pause"=w325) -> ("error out"=w335:errorcluster, "Elapsed?"=w327:bool, "Elapsed TIme"=w330:dbl)  [unwired: 6 in]
                n104 = Not(x=w325) -> (.not. x?=w329:bool)
                n105 = Not(x=w327) -> (.not. x?=w326:bool)
                n106 = And(x=w325, y=w326) -> (x .and. y?=w328:bool)
                n107 = Bundle By Name(cluster=w340, "Car Wash Indicators.Vehicle Out of Position"=w329, "Elapsed TIme"=w330, "Car Wash Indicators.Tire Shine Foam"=w328) -> (w339:T5)
                n108 = Select(t=T3 {"Command"=enum."Air Dry", "Data"=variant} ("Car wash cmd data cluster"), s=w327, f=T3 {"Command"=enum."Tire Shine Foam", "Data"=variant}) -> (s? t:f=w331:T3)
                n109 = Enqueue Element(queue=w337, element=w331, error in (no error)=w335) -> (error out=w338:errorcluster)  [unwired: 1 in, 2 out]
              }
              frame False {
                n110 = Bundle By Name(cluster=w348, "Wash Entry"=TRUE) -> (w347:T5)
                n111 = Enqueue Element(queue=w343, element=T3 {"Command"=enum."Air Dry", "Data"=variant} ("Car wash cmd data cluster"), error in (no error)=w342) -> (error out=w344:errorcluster)  [unwired: 1 in, 2 out]
              }
            }
          }
          frame "Air Dry" {
            w354 = u8 3 items=["Entry", "Station 1", "Station 2", "Station 3", "Exit"] ("Car Position Slider")
            n112 = Unbundle By Name(w353) -> ("Tire Shine Foam"=w352:bool)
            n113 = call "fgv.vi"("Command"=fgv."Get Car Pos.", "error in (no error)"=w358) -> ("error out"=w357:errorcluster, "Car Position Slider 2"=w355:u8)  [unwired: 8 in]
            n114 = Equal?(x=w354, y=w355) -> (x = y?=w351:bool)
            n115 = case shown="True" w352 {
              tunnel: w362 -> [w379 w387]
              tunnel: [w378 w386] -> w361
              tunnel: [w377 w383] -> w360
              tunnel: w359 -> [w376 w382]
              tunnel: w357 -> [w375 w381]
              tunnel: w351 -> [w364 _]
              tunnel: w350 -> [w373 _]
              tunnel: [w366 TRUE ("Elapsed?")] -> w349
              frame True {
                n116 = call "Timer.vi"("error in (no error)"=w375, "Reset"=w373, "Pause"=w364) -> ("error out"=w374:errorcluster, "Elapsed?"=w366:bool, "Elapsed TIme"=w369:dbl)  [unwired: 6 in]
                n117 = Not(x=w364) -> (.not. x?=w368:bool)
                n118 = Not(x=w366) -> (.not. x?=w365:bool)
                n119 = And(x=w364, y=w365) -> (x .and. y?=w367:bool)
                n120 = Bundle By Name(cluster=w379, "Car Wash Indicators.Vehicle Out of Position"=w368, "Elapsed TIme"=w369, "Car Wash Indicators.Air Dry"=w367) -> (w378:T5)
                n121 = Select(t=T3 {"Command"=enum."Air Dry", "Data"=variant} ("Car wash cmd data cluster"), s=w366, f=T3 {"Command"=enum."Air Dry", "Data"=variant}) -> (s? t:f=w370:T3)
                n122 = Enqueue Element(queue=w376, element=w370, error in (no error)=w374) -> (error out=w377:errorcluster)  [unwired: 1 in, 2 out]
              }
              frame False {
                n123 = Bundle By Name(cluster=w387, "Wash Entry"=TRUE) -> (w386:T5)
                n124 = Enqueue Element(queue=w382, element=T3 {"Command"=enum."Air Dry", "Data"=variant} ("Car wash cmd data cluster"), error in (no error)=w381) -> (error out=w383:errorcluster)  [unwired: 1 in, 2 out]
              }
            }
          }
          frame "Stop" {
            w391 = u8 0 items=["Entry", "Station 1", "Station 2", "Station 3", "Exit"] ("Car Position Slider")
            (unwired) FALSE
            # "Reinitializing all the controls and \nindicator to its default value"
            # "This case Stop the VI and Reinitializing all the controls and \nindicator to its default value."
            n125 = local write "Wash Options"(T1 {"Underbody Wash"=FALSE, "Bug Remover"=FALSE, "Pre-Soak"=FALSE, "High Pressure Wash"=FALSE, "Low Pressure Wax"=FALSE, "Spot Free Rinse"=FALSE, "Tire Shine Foam"=FALSE, "Air Dry"=FALSE} ("Wash Options")) -> ()
            n126 = local write "Car Position Slider"(w391) -> ()
          }
        }
        n127 = Unbundle By Name(w33) -> ("Car Wash Indicators"=→"Car Wash Indicators":T2, "Wash Entry"=→"Wash Entry":bool, "Elapsed TIme"=→"Elapsed Time":dbl)
        n128 = Unbundle By Name(w36) -> ("status"=w38:bool)
        n129 = Or(x=w38, y=w37) -> (x .or. y?=w35:bool)
      }
      frame Error {
        # "If there is error then this case will execute and it will stop the VI"
      }
    }
    n130 = Wait (ms)(milliseconds to wait=u32 100) -> ()  [unwired: 1 out]
  }
  n131 = while {
    shift-right: [w402] -> w5
    shift-left: w11 -> [w404]
    tunnel: w10 -> [w405]
    stop <- w403 stop-if-true
    n132 = event shown="[2] \"Car Position Slider\": Value Change" {
      selector: _ -> [_ _ _]
      dyn-events: _ -> [_ _ _]
      timeout: _ -> [_ _ _]
      tunnel: w405 -> [w413 w418 _]
      tunnel: w404 -> [w412 w417 w423]
      tunnel: [w411 w416 w422] -> w402
      tunnel: [FALSE TRUE FALSE] -> w400
      event "Start": Value Change {
        n133 = event-data() -> ()  [unwired: 1 in, 1 out]
        n134 = To Variant(anything="Wash Options") -> (Variant=w407:variant)
        n135 = Bundle By Name(cluster=T3 {"Command"=enum."Start", "Data"=variant} ("Car wash cmd data cluster"), "Data"=w407) -> (w406:T3)
        n136 = Enqueue Element(queue=w413, element=w406, error in (no error)=w412) -> (error out=w411:errorcluster)  [unwired: 1 in, 2 out]
      }
      event "stop": Value Change {
        n137 = event-data() -> ()  [unwired: 1 in, 1 out]
        n138 = Enqueue Element(queue=w418, element=T3 {"Command"=enum."Stop", "Data"=variant} ("Car wash cmd data cluster"), error in (no error)=w417) -> (error out=w416:errorcluster)  [unwired: 1 in, 2 out]
      }
      event "Car Position Slider": Value Change {
        n139 = event-data() -> ()  [unwired: 1 in, 1 out]
        n140 = call "fgv.vi"("Command"=fgv."Set Car Pos.", "error in (no error)"=w423, "Car Position Slider"="Car Position Slider") -> ("error out"=w422:errorcluster)  [unwired: 7 in, 1 out]
      }
    }
    n141 = Unbundle By Name(w402) -> ("status"=w401:bool)
    n142 = Or(x=w401, y=w400) -> (x .or. y?=w403:bool)
  }
  n143 = Merge Errors(w5, w3) -> (w4:errorcluster)
  n144 = Release Queue(queue=w10, error in (no error)=w4) -> (error out=w2:errorcluster)  [unwired: 1 in, 2 out]
  n145 = call <vilib>:"Simple Error Handler.vi"("error in (no error)"=w2) -> ()  [unwired: 4 in, 5 out]
